vi "build menu.vi"(8 "error in (no error)":errorcluster, 11 "UI elements cluster":T1) -> (0 "error out":errorcluster, 3 "UI elements cluster":T1)   [LabVIEW 2020]
uses:
  Typedefs/UI ctrl refs cluster.ctl
  Typedefs/Laser control knob.ctl
  Typedefs/Frame Size.ctl
  Typedefs/Plane Mode.ctl
  Typedefs/PMT control knob.ctl
  Typedefs/XY Stage_Move.ctl
  Typedefs/test_fpga_control.ctl
  Acquisition/Typedefs/Ref DAQ Param.ctl
  Misc/Experiment Type.ctl
  Misc/Biology Information.ctl
  <vilib>/Utility/miscctls.llb/LVMenuShortCut.ctl
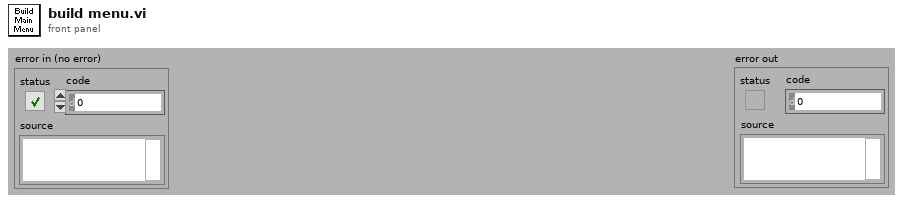
[diagram p1: front panel]
types:
  T1 = typedef "UI ctrl refs cluster.ctl" = cluster{"Top level VI path":path, "Top level VI ref":refnum<vi>, "User menu ref":refnum<k9>, "Sub Panel control":refnum<vi>, "Imaging Param Tab":refnum<vi>, "Occurrence-Start drivers":refnum<k4>, "Occurrence-Speed logging initialised":refnum<k4>, "Occurrence-XYZ stage initialised":refnum<k4>, "Exit button":refnum<vi>, "Status ind":refnum<vi>, "Set as origin":refnum<vi>, "Speed Logging":refnum<vi>, "Time Lapse":refnum<vi>, "Live Imaging":refnum<vi>, "AOL Z Stack":refnum<vi>, "Motor Z Stack":refnum<vi>, "Funct Acq button":refnum<vi>, "Hard Shutter":refnum<vi>, "Virtual Shutter":refnum<vi>, "Laser Power":refnum<vi>, "AOL Mode":refnum<vi>, "Frame Size":refnum<vi>, "Field of View":refnum<vi>, "Dwell Time":refnum<vi>, "Zoom":refnum<vi>, "AOL Z":refnum<vi>, "Objective":refnum<vi>, "Axis":refnum<vi>, "Paths & Names":refnum<vi>, "Experiment folder path (ind.)":refnum<vi>, "Last State (Ind.)":refnum<vi>, "Averages":refnum<vi>, "Angle (degrees)":refnum<vi>, "X centre":refnum<vi>, "Y centre":refnum<vi>, "Plane Mode":refnum<vi>, "# Planes":refnum<vi>, "Z Start":refnum<vi>, "Z Stop":refnum<vi>, "Z Step":refnum<vi>, "PMT 1":refnum<vi>, "PMT 2":refnum<vi>, "Stage XYZ Position":refnum<vi>, "Pockels@Z Start":refnum<vi>, "Pockels@Z Stop":refnum<vi>, "Obtain Z Start":refnum<vi>, "Obtain Z Stop":refnum<vi>, "Live stim.trig.period":refnum<vi>, "Live stim.trig.enable":refnum<vi>, "Movement Correction":refnum<vi>, "Load Reference Image":refnum<vi>, "XY Stage Move":refnum<vi>, "MovCor Cluster":refnum<vi>, "RefDAQParam":refnum<vi>, "Funct. Acq. Pockels Modulation":refnum<vi>, "Ref Laser Power":refnum<vi>, "Enable Video Recording":refnum<vi>, "Video Record-Live Imaging":refnum<vi>, "Video Record-Funct acq":refnum<vi>, "Reference Source":refnum<vi>, "AOL Z-stack Chirps Ready (ind)":refnum<vi>, "Target time between mov.cor. ref triggers (ms)":refnum<vi>, "Funct. Acq. Ref frame save":refnum<vi>, "Tracking button":refnum<vi>, "Show ref plots window":refnum<vi>, "Center freq ind (nm)":refnum<vi>, "Pickup mode (ind)":refnum<vi>, "Logging queue (ind)":refnum<vi>, "Back aperture power (ind.)":refnum<vi>, "Power after objective (ind.)":refnum<vi>, "Switch user":refnum<vi>, "Ls1 Conn. Status":refnum<vi>, "Ls1Tuning Status":refnum<vi>, "Ls1 Faults":refnum<vi>, "Ls1 Connection":refnum<vi>, "Ls1 Mode":refnum<vi>, "Ls1 POWER [mW]":refnum<vi>, "Ls1Shutter":refnum<vi>, "Ls1 Wavelength":refnum<vi>, "Ls1 Note":refnum<vi>, "Ls1 Confirm Wav":refnum<vi>, "Ls1 PreChrp Prism1":refnum<vi>, "Ls1 PreChrp Prism2":refnum<vi>, "Ls1 wav top Ind":refnum<vi>, "Ls1 power top Ind":refnum<vi>, "Ls1 Pump peak Hold":refnum<vi>, "Ls1 Status Ind":refnum<vi>, "Ls1 wav cancel":refnum<vi>, "Experiment Type":refnum<vi>, "Biology Information":refnum<vi>, "Camera recording status":refnum<vi>, "Optimise Obj. Pos.":refnum<vi>}
  T2 = typedef "LVMenuShortCut.ctl" = cluster{"Include Shift Key?":bool, "Include Ctrl Key?":bool, "Shortcut Key":string}
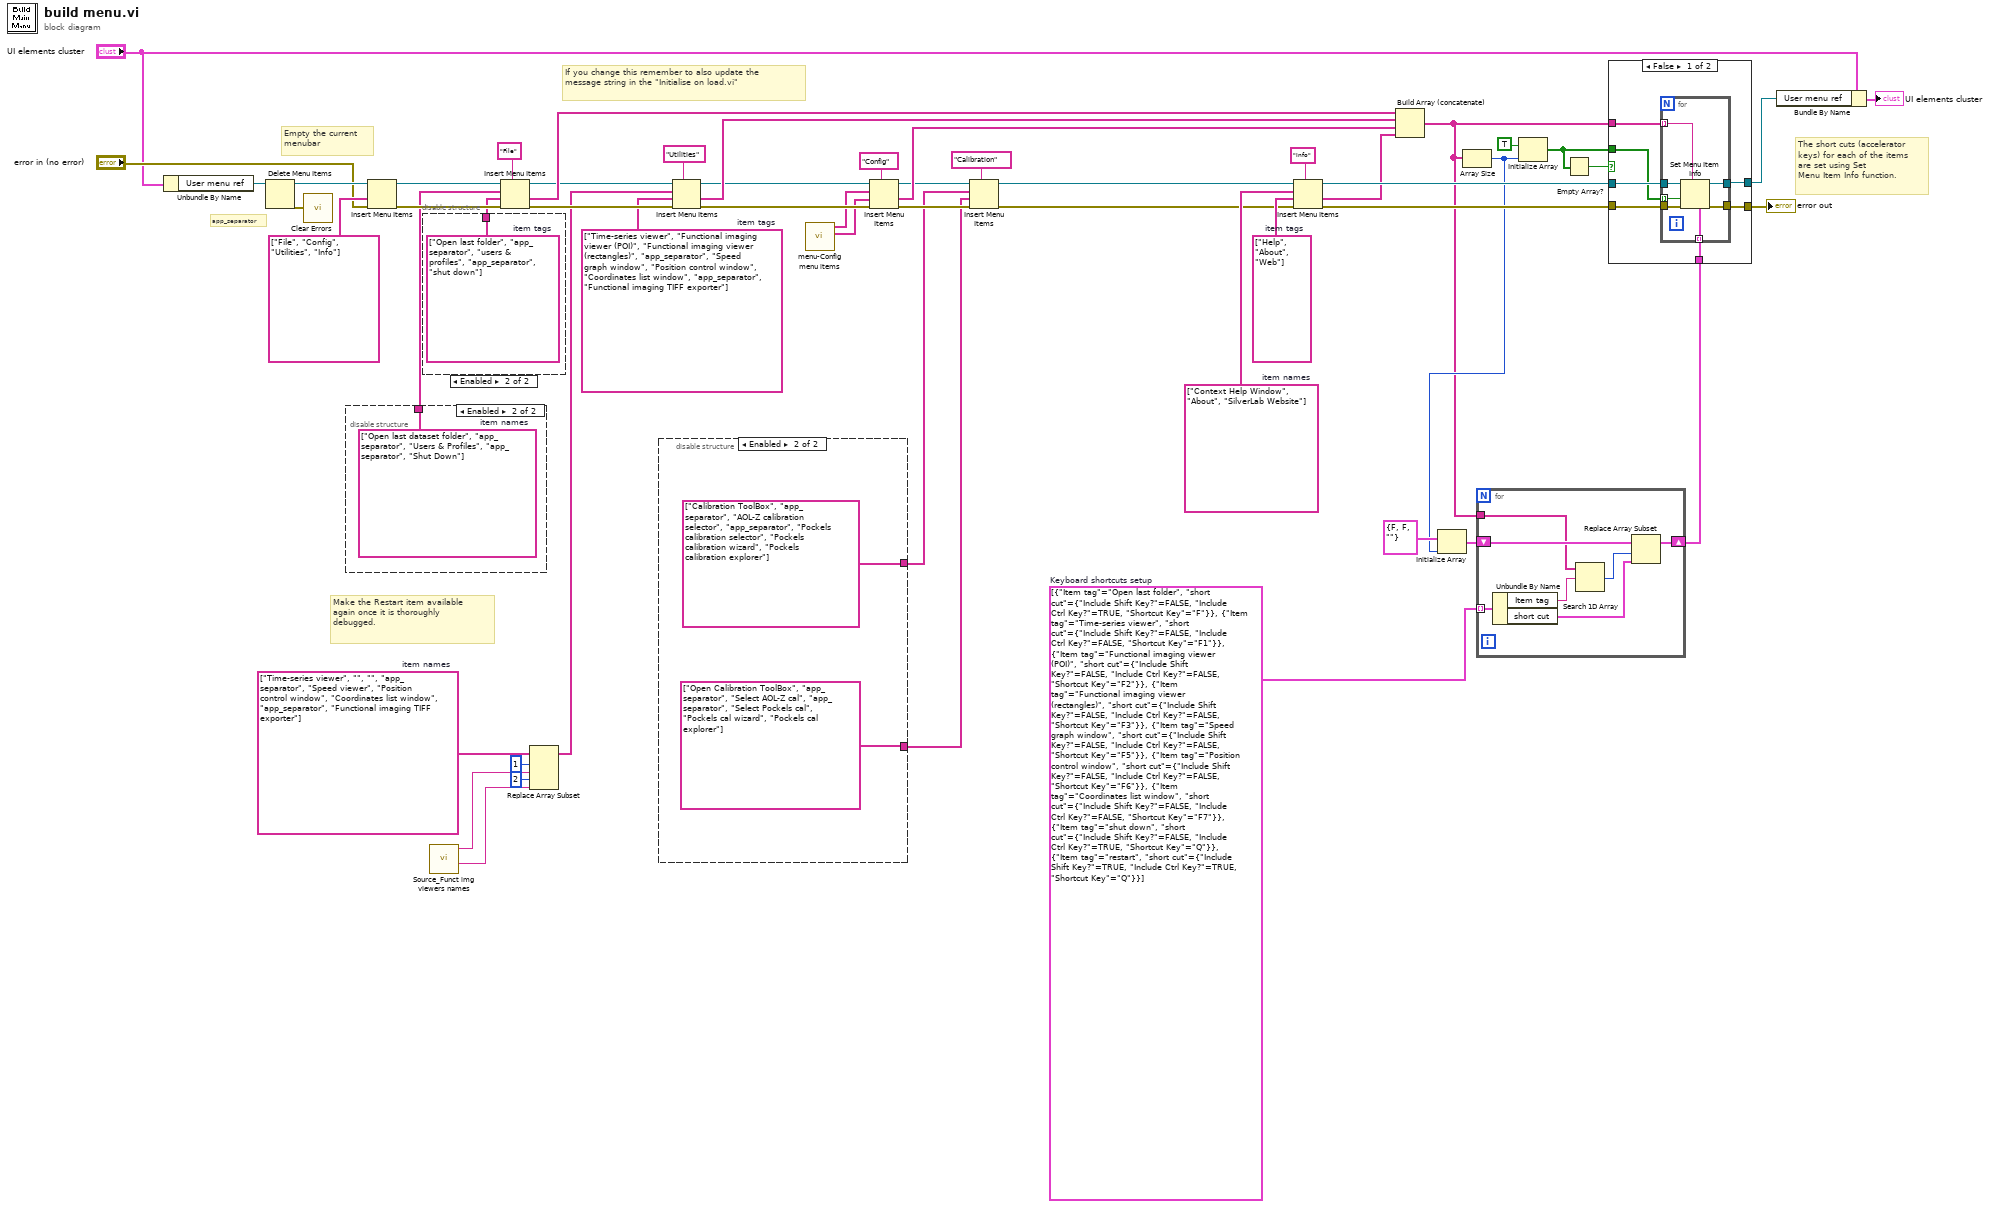
[diagram p0: block diagram]
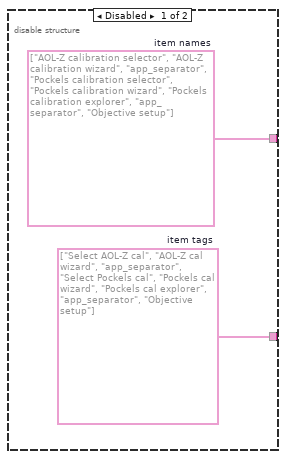
[diagram p2: hidden frame]
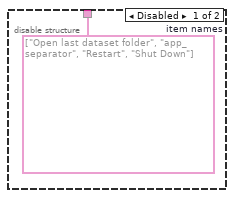
[diagram p4: hidden frame]
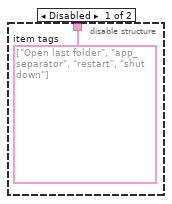
[diagram p5: hidden frame]
diagram:
  w7 = string[] ["Time-series viewer", "Functional imaging viewer (POI)", "Functional imaging viewer (rectangles)", "app_separator", "Speed graph window", "Position control window", "Coordinates list window", "app_separator", "Functional imaging TIFF exporter"]  # item tags
  w6 = string[] ["Time-series viewer", "", "", "app_separator", "Speed viewer", "Position control window", "Coordinates list window", "app_separator", "Functional imaging TIFF exporter"]  # item names
  w16 = cluster{"Item tag":string, "short cut":T2}[] [{"Item tag"="Open last folder", "short cut"={"Include Shift Key?"=FALSE, "Include Ctrl Key?"=TRUE, "Shortcut Key"="F"}}, {"Item tag"="Time-series viewer", "short cut"={"Include Shift Key?"=FALSE, "Include Ctrl Key?"=FALSE, "Shortcut Key"="F1"}}, {"Item tag"="Functional imaging viewer (POI)", "short cut"={"Include Shift Key?"=FALSE, "Include Ctrl Key?"=FALSE, "Shortcut Key"="F2"}}, {"Item tag"="Functional imaging viewer (rectangles)", "short cut"={"Include Shift Key?"=FALSE, "Include Ctrl Key?"=FALSE, "Shortcut Key"="F3"}}, {"Item tag"="Speed graph window", "short cut"={"Include Shift Key?"=FALSE, "Include Ctrl Key?"=FALSE, "Shortcut Key"="F5"}}, {"Item tag"="Position control window", "short cut"={"Include Shift Key?"=FALSE, "Include Ctrl Key?"=FALSE, "Shortcut Key"="F6"}}, {"Item tag"="Coordinates list window", "short cut"={"Include Shift Key?"=FALSE, "Include Ctrl Key?"=FALSE, "Shortcut Key"="F7"}}, {"Item tag"="shut down", "short cut"={"Include Shift Key?"=FALSE, "Include Ctrl Key?"=TRUE, "Shortcut Key"="Q"}}, {"Item tag"="restart", "short cut"={"Include Shift Key?"=TRUE, "Include Ctrl Key?"=TRUE, "Shortcut Key"="Q"}}]  # Keyboard shortcuts setup
  w35 = string[] ["Context Help Window", "About", "SilverLab Website"]  # item names
  w37 = string[] ["Help", "About", "Web"]  # item tags
  # "If you change this remember to also update the message string in the \"Initialise on load.vi\""
  # "Make the Restart item available again once it is thoroughly debugged."
  # "app_separator"
  # "Empty the current\nmenubar"
  # "The short cuts (accelerator\nkeys) for each of the items\nare set using Set\nMenu Item Info function."
  n1 = Unbundle By Name("UI elements cluster") -> ("User menu ref"=w13:refnum<k9>)
  n2 = Delete Menu Items(9:w13) -> (0:w43:errorcluster, 3:w50:refnum<k9>)  [unwired: 2 in, 1 out]
  n3 = call <vilib>:"Clear Errors.vi"("error in (no error)"=w43) -> ()  [unwired: 5 in, 2 out]
  n4 = disable-structure shown="Enabled" {
    disable-tunnel: [w55 w56] -> w23
    frame Disabled {
      w55 = string[] ["Open last dataset folder", "app_separator", "Restart", "Shut Down"]  # item names
    }
    frame Enabled {
      w56 = string[] ["Open last dataset folder", "app_separator", "Users & Profiles", "app_separator", "Shut Down"]  # item names
    }
  }
  n5 = Insert Menu Items(6:"error in (no error)", 7:string[] ["File", "Config", "Utilities", "Info"] ("item tags"), 9:w50) -> (0:w51:errorcluster, 3:w44:refnum<k9>)  [unwired: 4 out]
  n6 = disable-structure shown="Enabled" {
    disable-tunnel: [w57 w58] -> w48
    frame Disabled {
      w57 = string[] ["Open last folder", "app_separator", "restart", "shut down"]  # item tags
    }
    frame Enabled {
      w58 = string[] ["Open last folder", "app_separator", "users & profiles", "app_separator", "shut down"]  # item tags
    }
  }
  n7 = call "Source_Funct img viewers names.vi"() -> ("Name string: Functional imaging viewer (Rectangles)"=w2:string, "Name string: Functional imaging viewer (POI/Mscn)"=w1:string)  [unwired: 10 in]
  n8 = Insert Menu Items(5:"File" ("menu tag"), 6:w51, 7:w48, 8:w23, 9:w44) -> (0:w52:errorcluster, 1:w49:string[], 3:w45:refnum<k9>)  [unwired: 1 out]
  n9 = Replace Array Subset(array=w6, new element #1=w1, index #1=1 ("index"), new element #2=w2, index #2=2 ("index")) -> (w4:string[])
  n10 = disable-structure shown="Enabled" {
    disable-tunnel: [w60 string[] ["Open Calibration ToolBox", "app_separator", "Select AOL-Z cal", "app_separator", "Select Pockels cal", "Pockels cal wizard", "Pockels cal explorer"] ("item names")] -> w26
    disable-tunnel: [w59 string[] ["Calibration ToolBox", "app_separator", "AOL-Z calibration selector", "app_separator", "Pockels calibration selector", "Pockels calibration wizard", "Pockels calibration explorer"] ("item names")] -> w22
    frame Disabled {
      w59 = string[] ["AOL-Z calibration selector", "AOL-Z calibration wizard", "app_separator", "Pockels calibration selector", "Pockels calibration wizard", "Pockels calibration explorer", "app_separator", "Objective setup"]  # item names
      w60 = string[] ["Select AOL-Z cal", "AOL-Z cal wizard", "app_separator", "Select Pockels cal", "Pockels cal wizard", "Pockels cal explorer", "app_separator", "Objective setup"]  # item tags
    }
    frame Enabled {
    }
  }
  n11 = Insert Menu Items(5:"Utilities" ("menu tag"), 6:w52, 7:w7, 8:w4, 9:w45) -> (0:w24:errorcluster, 1:w40:string[], 3:w25:refnum<k9>)  [unwired: 1 out]
  n12 = call "menu-Config menu items.vi"() -> ("item tags"=w14:string[], "item names"=w15:string[])  [unwired: 10 in]
  n13 = Insert Menu Items(5:"Config", 6:w24, 7:w14, 8:w15, 9:w25) -> (0:w30:errorcluster, 1:w38:string[], 3:w31:refnum<k9>)  [unwired: 1 out]
  n14 = Insert Menu Items(5:"Calibration", 6:w30, 7:w26, 8:w22, 9:w31) -> (0:w29:errorcluster, 3:w28:refnum<k9>)  [unwired: 2 out]
  n15 = Insert Menu Items(5:"Info" ("menu tag"), 6:w29, 7:w37, 8:w35, 9:w28) -> (0:w53:errorcluster, 1:w36:string[], 3:w47:refnum<k9>)  [unwired: 1 out]
  n16 = Build Array (concatenate)(w49, w40, w38, w36) -> (w17:string[])
  n17 = Array Size(array=w17) -> (size(s)=w18:i32)
  n18 = Initialize Array(T2 {"Include Shift Key?"=FALSE, "Include Ctrl Key?"=FALSE, "Shortcut Key"=""} ("short cut"), w18) -> (w19:T2[])
  n19 = for {
    shift-right: [w69] -> w20
    shift-left: w19 -> [w68]
    tunnel: w16 -> [w67] mode=indexing
    tunnel: w17 -> [w65]
    n20 = Unbundle By Name(w67) -> ("Item tag"=w64:string, "short cut"=w66:T2)
    n21 = Search 1D Array(1D array=w65, element=w64) -> (index of element=w63:i32)  [unwired: 1 in]
    n22 = Replace Array Subset(array=w68, new element=w66, index=w63) -> (w69:T2[])
  }
  n23 = Initialize Array(TRUE, w18) -> (w9:bool[])
  n24 = Empty Array?(array=w9) -> (empty?=w8:bool)
  n25 = case shown="False" w8 {
    tunnel: [w76 w84] -> w54
    tunnel: w53 -> [w75 w84]
    tunnel: w47 -> [w74 w85]
    tunnel: w20 -> [w73 _]
    tunnel: w17 -> [w72 _]
    tunnel: [w71 w85] -> w11
    tunnel: w9 -> [w70 _]
    frame False {
      n26 = for {
        tunnel: w74 -> [w83]
        tunnel: [w82] -> w71
        tunnel: w72 -> [w81] mode=indexing
        tunnel: w75 -> [w80]
        tunnel: [w79] -> w76
        tunnel: w70 -> [w78] mode=indexing
        tunnel: w73 -> [w77] mode=indexing
        n27 = Set Menu Item Info(4:w77, 7:w81, 8:w80, 9:w78, 11:w83) -> (0:w79:errorcluster, 3:w82:refnum<k9>)  [unwired: 2 out]
      }
    }
    frame True {
      # "Fail-safe case"
    }
  }
  "error out" <- w54
  n28 = Bundle By Name(cluster="UI elements cluster", "User menu ref"=w11) -> (→"UI elements cluster":T1)
